vi "ROI group-Modify ROI Group.vi"(8 "error in (no error)":errorcluster, 11 "Save? (T)":bool=TRUE) -> (0 "error out":errorcluster, 1 "New group setup":T1 {"Group region specifier cluster"."Contours"."Type" items=["No Selection", "Point", "Line", "Rectangle", "Oval", "Polygon", "Freehand Region", "Annulus", "Unused2", "Unused3", "Broken Line", "Freehand Line", "Rotated Rectangle"]}, 3 "Cancelled or Error":bool)   [LabVIEW 2020]
uses:
  ROI Selection Interface/ROI group info cluster.ctl
  Experiment header interface/Typedefs/Save-Load-Save as-Load last enum.ctl
  Global variables/gl_Functional Imaging-Global variables.vi
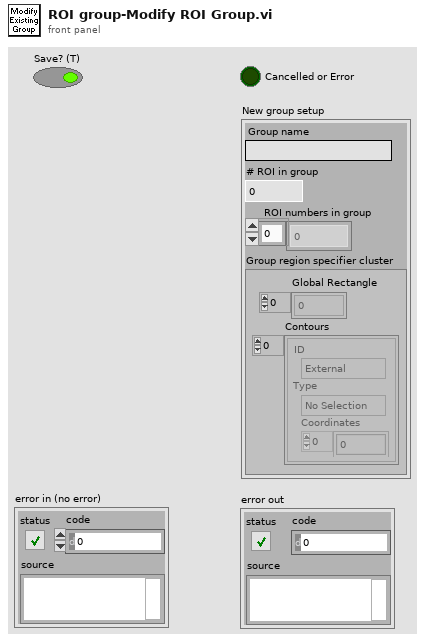
[diagram p1: front panel]
types:
  T1 = typedef "ROI group info cluster.ctl" = cluster{"Group name":string, "# ROI in group":i32, "ROI numbers in group":i32[], "Group region specifier cluster":T2}
  T2 = typedef "ROI Descriptor" = cluster{"Global Rectangle":i32[], "Contours":cluster{"ID":enum32{"External", "Internal"}, "Type":u32, "Coordinates":i32[]}[]}
  T3 = typedef "Functional Imging UI Refs.ctl" = cluster{"Menu ref":refnum<k9>, "Image control":refnum<vi>, "VI ref":refnum<vi>, "XGrapher":refnum<vi>, "Smoothing":refnum<vi>, "POI Averaging":refnum<vi>, "Normalize":refnum<vi>, "POI data points in each trial":refnum<vi>, "Channel":refnum<vi>, "Experiment data folder path":refnum<vi>, "[ROI vis]":refnum<vi>, "[Groups] visbl":T4, "Group Name":refnum<vi>, "POI index":refnum<vi>, "Trial No.":refnum<vi>, "Intensity Zoom":refnum<vi>, "Trial Cursor Enabled":refnum<vi>, "Number of Trials (ind 1)":refnum<vi>, "Number of Trials (ind 2)":refnum<vi>, "MiniScans Available":refnum<vi>, "POI Available":refnum<vi>, "Defer graph updates":refnum<vi>, "Waveform selector":refnum<vi>, "#of selected POI":refnum<vi>, "#of selected MiniScans":refnum<vi>, "#of selected groups":refnum<vi>, "Max Z-Projection":refnum<vi>, "Z-Plane Selector":refnum<vi>, "Index of miniscan point to visualise":refnum<vi>, "ROI vis. mode":refnum<vi>, "Total # of points":refnum<vi>, "Index of group clicked on":refnum<vi>, "Pane 1":refnum<vi>, "Pane 2":refnum<vi>, "Pane 3":refnum<vi>, "Pane 4":refnum<vi>, "Pane 5":refnum<vi>, "Pane 6":refnum<vi>, "Deselect all ROI":refnum<vi>, "Deselect all groups":refnum<vi>}
  T4 = typedef "Groups array referecne.ctl" = refnum<vi>
  T5 = typedef "Save-Load-Save as-Load last enum.ctl" = enum16{"Save file", "Save file as", "Load file", "Load last file"}
  T6 = enum8{"Enabled", "Disabled", "Disabled and Grayed Out"}
  T7 = typedef "Group sel cluster.ctl" = cluster{"Group number":string, "Group Name":string, "Visibility":bool, "Highlight":bool}
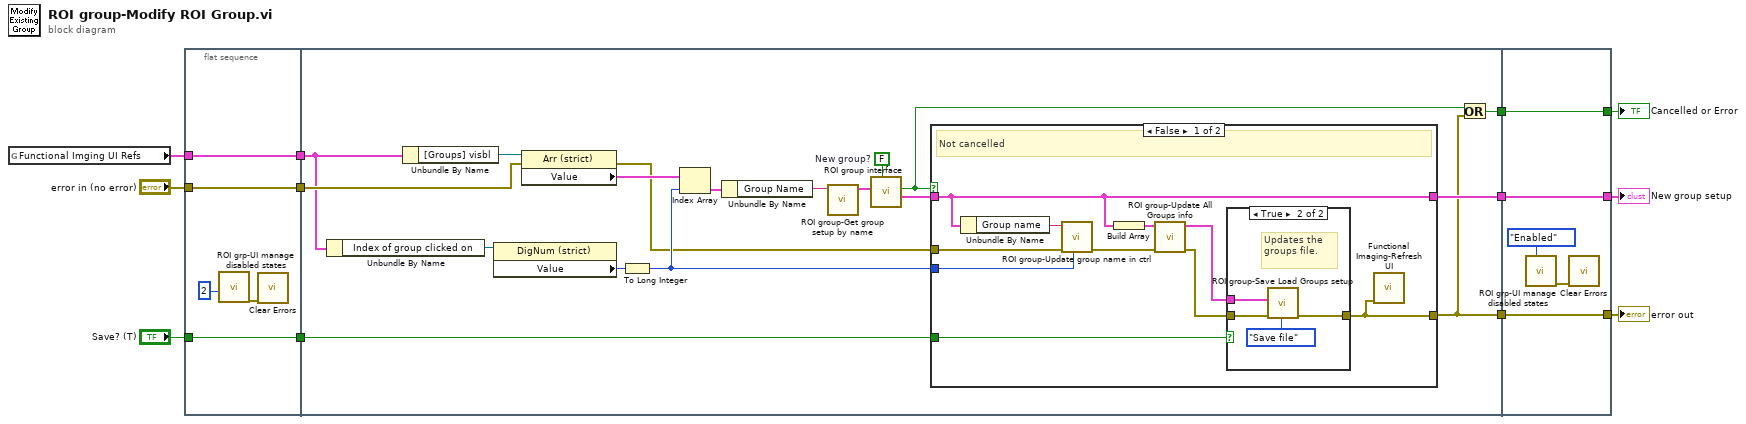
[diagram p0: block diagram]
diagram:
  n1 = global read "gl_Functional Imaging-Global variables.vi" "Functional Imging UI Refs"() -> (w9:T3)
  n2 = flat-sequence {
    tunnel: w9 -> [w16]
    tunnel: "error in (no error)" -> [w17]
    tunnel: [w17] -> w4
    tunnel: [w16] -> w3
    tunnel: [w13] -> w2
    tunnel: "Save? (T)" -> [w13]
    tunnel: [w35] -> w7
    tunnel: [w34] -> w6
    tunnel: [w22] -> w5
    tunnel: w4 -> [w32]
    tunnel: w3 -> [w23]
    tunnel: w2 -> [w18]
    tunnel: [w54] -> w8
    tunnel: [w55] -> w11
    tunnel: [w56] -> w12
    tunnel: w7 -> [w56]
    tunnel: w6 -> [w55]
    tunnel: w5 -> [w54]
    frame #0 {
      n3 = call "ROI grp-UI manage disabled states.vi"("UI elemente enabled?"=2) -> ("error out"=w14:errorcluster)  [unwired: 10 in]
      n4 = call <vilib>:"Clear Errors.vi"("error in (no error)"=w14) -> ()  [unwired: 5 in, 2 out]
    }
    frame #1 {
      w27 = FALSE  # New group?
      n5 = Unbundle By Name(w23) -> ("Index of group clicked on"=w25:refnum<vi>)
      n6 = Unbundle By Name(w23) -> ("[Groups] visbl"=w33:T4)
      n7 = property on="Property Node" class="DigNum (strict)"(reference=w25) -> ("Value"=w24:i16)  [unwired: 1 in, 2 out]
      n8 = property on="Property Node" class="Arr (strict)"(reference=w33, error in=w32) -> (error out=w21:errorcluster, "Value"=w31:T7[])  [unwired: 1 out]
      n9 = To Long Integer(number=w24) -> (32bit integer=w26:i32)
      n10 = Index Array(array=w31, index=w26) -> (element=w30:T7)
      n11 = Unbundle By Name(w30) -> ("Group Name"=w20:string)
      n12 = call "ROI group-Get group setup by name.vi"("Name of ROI group to search for"=w20) -> ("POI group info cluster"=w19:T1)  [unwired: 8 in, 2 out]
      n13 = call "ROI group interface.vi"("New group (F)"=w27, "POI group info cluster in"=w19) -> ("POI group info cluster"=w29:T1, "Cancelled"=w28:bool)  [unwired: 7 in, 1 out]
      n14 = case shown="False" w28 {
        tunnel: w29 -> [w45 _]
        tunnel: [w39 w51] -> w22
        tunnel: [w45 _] -> w35
        tunnel: w26 -> [w43 _]
        tunnel: w21 -> [w40 w51]
        tunnel: w18 -> [w36 _]
        frame False {
          # "Not cancelled"
          n15 = Unbundle By Name(w45) -> ("Group name"=w44:string)
          n16 = call "ROI group-Update group name in ctrl.vi"("Index of group to update"=w43, "error in (no error)"=w40, "Group Name"=w44) -> ("error out"=w41:errorcluster)  [unwired: 8 in]
          n17 = Build Array(w45) -> (w42:T1[])
          n18 = call "ROI group-Update All Groups info.vi"("error in (no error)"=w41, "Groups setup to add/update"=w42) -> ("error out"=w38:errorcluster, "Updated \"All groups\" setup"=w37:T1[])  [unwired: 8 in]
          n19 = case shown="True" w36 {
            tunnel: w38 -> [w46 w49]
            tunnel: w37 -> [_ w48]
            tunnel: [w46 w47] -> w39
            frame False {
            }
            frame True {
              # "Updates the groups file."
              n20 = call "ROI group-Save Load Groups setup.vi"("error in (no error)"=w49, "Function"=Save-Load-Save_as-Load_last_enum."Save file", "Groups setup to save"=w48) -> ("error out"=w47:errorcluster)  [unwired: 7 in, 1 out]
            }
          }
          n21 = call "Functional Imaging-Refresh UI.vi"("error in (no error)"=w39) -> ()  [unwired: 11 in]
        }
        frame True {
          # "Cancelled"
        }
      }
      n22 = Or(x=w28, y=w22) -> (x .or. y?=w34:bool)
    }
    frame #2 {
      n23 = call "ROI grp-UI manage disabled states.vi"("UI elemente enabled?"=T6."Enabled") -> ("error out"=w53:errorcluster)  [unwired: 10 in]
      n24 = call <vilib>:"Clear Errors.vi"("error in (no error)"=w53) -> ()  [unwired: 5 in, 2 out]
    }
  }
  "error out" <- w8
  "New group setup" <- w12
  "Cancelled or Error" <- w11
